vi "Convert Errors to MCL ItemNames.vi"(1 "Errors To Display":T1[](array[typedef])) -> (0 "ItemNames":string[][](array[string]))   [LabVIEW 2016, in "Error Manager.lvlib"]
doc: "Blank VI with error handling."
uses:
  Error Manager.lvlib
  Read-Unread Status (enum).ctl
  Handled Error (cluster).ctl
panel:
  # "Input\nInputs to the VI"
  # "Development\nControls or indicators that are useful for development or testing, but which are not outputs of the VI."
  # "Output\nOutputs of the VI"
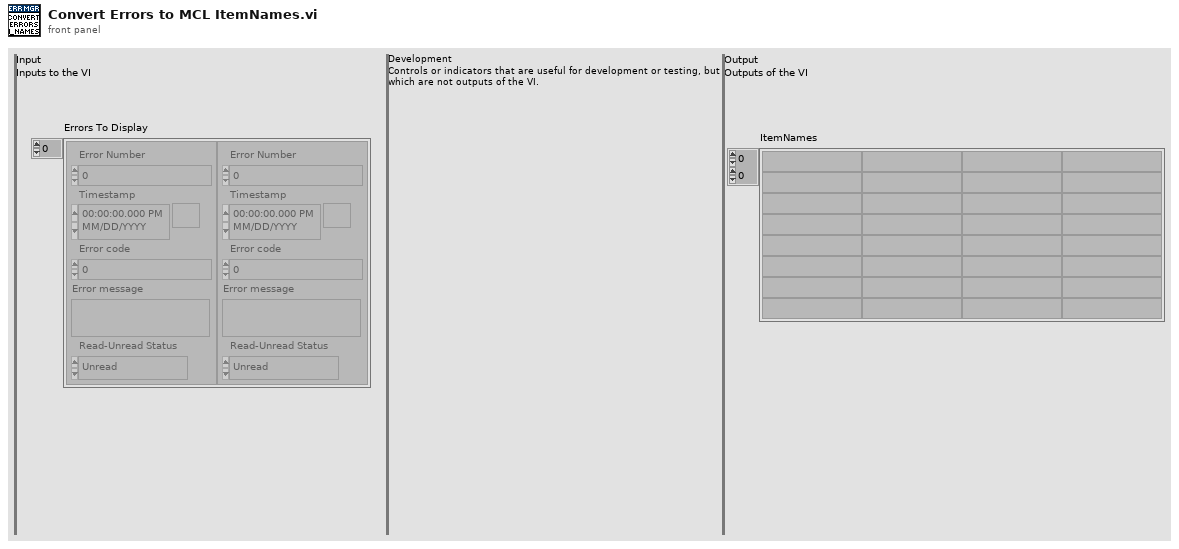
[diagram p1: front panel]
types:
  T1 = typedef "Error Manager.lvlib/Handled Error (cluster).ctl" = cluster{"Error Number":i32, "Timestamp":timestamp, "Error code":i32, "Error message":string, "Read-Unread Status":T2}
  T2 = typedef "Error Manager.lvlib/Read-Unread Status (enum).ctl" = enum16{"Unread", "Read"}
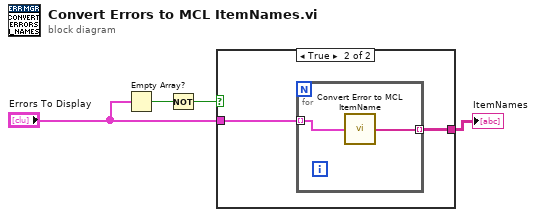
[diagram p0: block diagram]
diagram:
  n1 = Empty Array?(array="Errors To Display") -> (empty?=w4:bool)
  n2 = Not(x=w4) -> (.not. x?=w3:bool)
  n3 = case shown="True" w3 {
    tunnel: "Errors To Display" -> [_ w5]
    tunnel: [_ w6] -> w1
    frame False {
    }
    frame True {
      n4 = for {
        tunnel: w5 -> [w8] mode=indexing
        tunnel: [w7] -> w6 mode=indexing
        n5 = call "Convert Error to MCL ItemName.vi"("Error To Display"=w8) -> ("ItemName"=w7:string[])
      }
    }
  }
  "ItemNames" <- w1
